vi "Pin Position NumberLbcbs Write.vi"(4 "error in (no error)":errorcluster, 5 "Value":T2, 6 "Container State":T3, 7 "Display State In":T1) -> (0 "error out":errorcluster, 3 "Display State Out":T1)   [LabVIEW 2013, in "Pin Position.xctl"]
uses:
  Pin Position.xctl
  <vilib>/_xctls/Container State.ctl
  lib/Data Access Objects/Application/Number Of LBCBs.ctl
  Pin Position State.ctl
  <vilib>/_xctls/XControlSupport.lvlib
panel:
  # "Replace the Value Control below with a Control of desired type.\nDo not remove this Control or the others from the connector pane.\nDo not change the connector pane pattern.\nThe Value control should always be the third terminal from top on the input side in the connector pane."
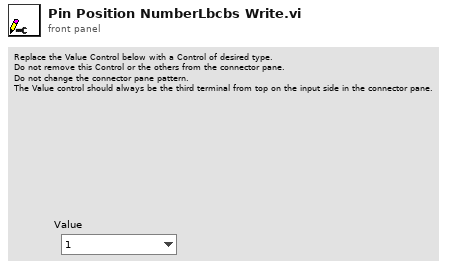
[diagram p1: front panel]
types:
  T1 = typedef "Pin Position.xctl/Pin Position State.ctl" = cluster{"Number  of LBCBs":T2, "RowNames":string[]}
  T2 = typedef "Number Of LBCBs.ctl" = enum16{"1", "2"}
  T3 = typedef "XControlSupport.lvlib/Container State.ctl" = cluster{"Indicator?":bool, "Run Mode?":bool, " Refnum":refnum<vi>}
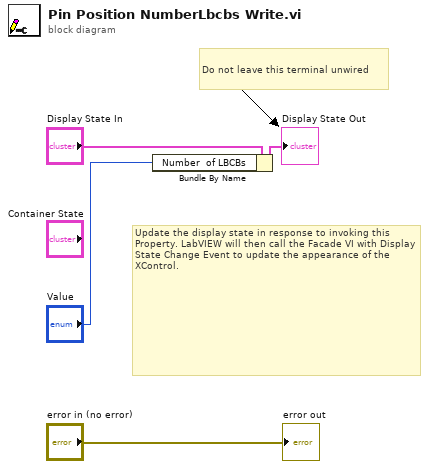
[diagram p0: block diagram]
diagram:
  # "Do not leave this terminal unwired"
  # "Update the display state in response to invoking this Property. LabVIEW will then call the Facade VI with Display State Change Event to update the appearance of the XControl."
  n1 = Bundle By Name(cluster="Display State In", "Number  of LBCBs"="Value") -> (→"Display State Out":T1)
  "error out" <- "error in (no error)"
